vi "Control Power Indicator Test.vi"(8 "error in (no error)":errorcluster, 10 "Message IN":string) -> (0 "error out":errorcluster, 1 "Result (bool)":bool, 2 "Message OUT":string)   [LabVIEW 2022 SP3]
panel:
  in  "stop":bool
  out "Instructional Message":string
  in  "OK Button":bool
  out "Result (color)":u32(colorbox)
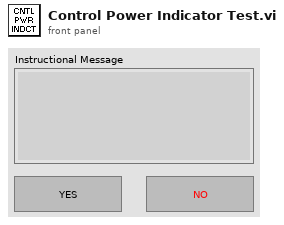
[diagram p1: front panel]
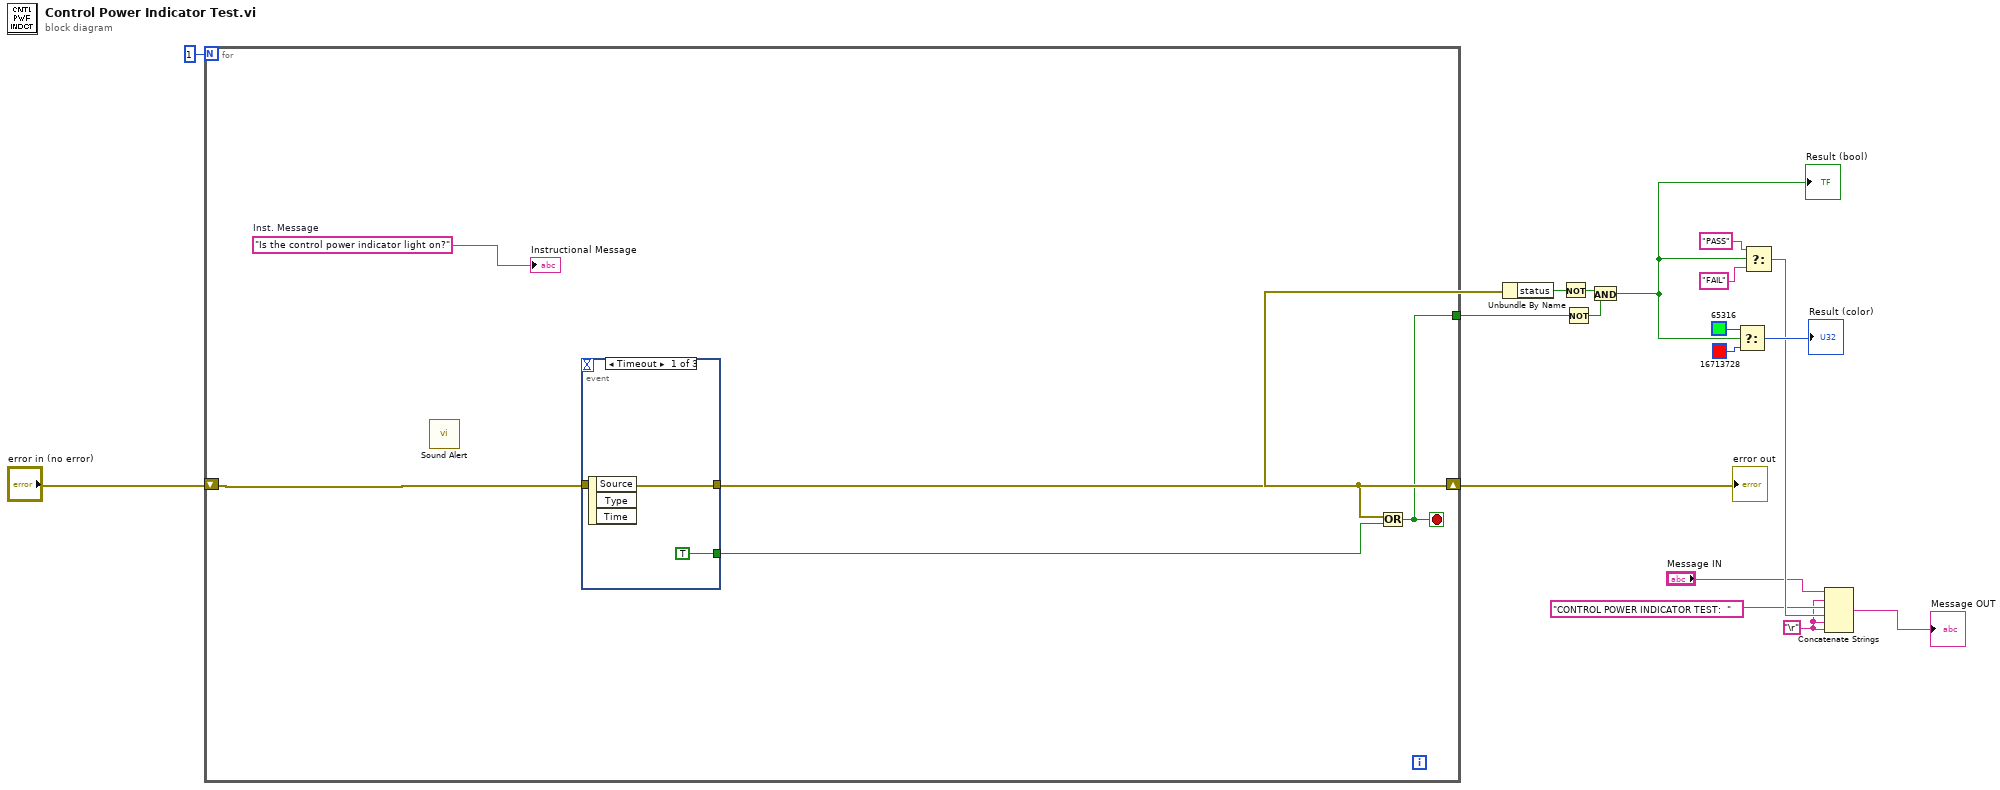
[diagram p0: block diagram]
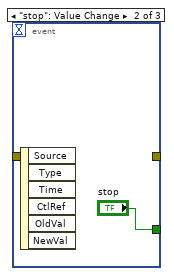
[diagram p2: hidden frame]
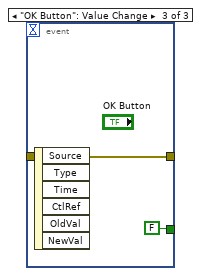
[diagram p3: hidden frame]
diagram:
  w3 = "\r"
  n1 = for {
    N: 1 -> [_]
    shift-right: [w23] -> w11
    shift-left: "error in (no error)" -> [w20]
    tunnel: [w21] -> w4
    stop <- w21 stop-if-true
    w19 = "Is the control power indicator light on?"  # Inst. Message
    n2 = call "Sound Alert.vi"() -> ()  [unwired: 12 in]
    n3 = event shown="[0] Timeout" {
      selector: _ -> [_ _ _]
      dyn-events: _ -> [_ _ _]
      timeout: _ -> [_ _ _]
      tunnel: w20 -> [w25 _ w28]
      tunnel: [w25 _ w28] -> w23
      tunnel: [TRUE "stop" FALSE] -> w22
      event Timeout {
        n4 = event-data() -> ()  [unwired: 1 in, 3 out]
      }
      event "stop": Value Change {
        n5 = event-data() -> ()  [unwired: 1 in, 6 out]
      }
      event "OK Button": Value Change {
        n6 = event-data() -> ()  [unwired: 1 in, 6 out]
      }
    }
    n7 = Or(x=w23, y=w22) -> (x .or. y?=w21:bool)
    "Instructional Message" <- w19
  }
  "error out" <- w11
  n8 = Unbundle By Name(w11) -> ("status"=w13:bool)
  n9 = Not(x=w13) -> (.not. x?=w12:bool)
  n10 = Not(x=w4) -> (.not. x?=w5:bool)
  n11 = And(x=w12, y=w5) -> (x .and. y?=w1:bool)
  "Result (bool)" <- w1
  n12 = Select(t=u32 65316 ("Result (color)"), s=w1, f=u32 16713728 ("Result (color)")) -> (s? t:f=→"Result (color)":u32)
  n13 = Select(t="PASS", s=w1, f="FAIL") -> (s? t:f=w9:string)
  n14 = Concatenate Strings("Message IN", w3, "CONTROL POWER INDICATOR TEST:  ", w9, w3, w3) -> (→"Message OUT":string)
